vi "FPGA_DMA_Init_5782.vi"(8 "error in (no error)":errorcluster, 11 "FPGA VI Reference":T1) -> (0 "error out":errorcluster, 3 "FPGA VI Out":T1, 5 "Remaining":u32)   [LabVIEW 2013]
uses:
  Config/FPGAref_5782_DMA.ctl
  <vilib>/rvi/interface/common/niFpgaWaitOnOcc.vi
  <vilib>/Utility/error.llb/Error Cluster From Error Code.vi
  <vilib>/rvi/errors/niLvFpgaAdjustHostInterfaceError.vi
  <vilib>/rvi/interface/nirviMethod/nirviMethod.xnode
  <vilib>/rvi/errors/niLvFpgaMergeErrorWithErrorCode.vi
  <vilib>/FPGAPlugInAG/Dynamic/niLvFpga_ReadFifo_Dynamic.vi
  <vilib>/FPGAPlugInAG/Dynamic/niLvFpga_ConfigureFifo_Dynamic.vi
  <vilib>/FPGAPlugInAG/Dynamic/niLvFpga_StartFifo_Dynamic.vi
panel:
  out "Actual Depth":u32
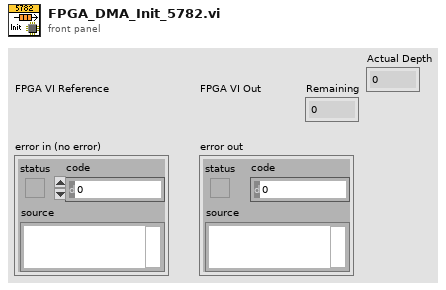
[diagram p1: front panel]
types:
  T1 = typedef "FPGAref_5782_DMA.ctl" = refnum<k20>
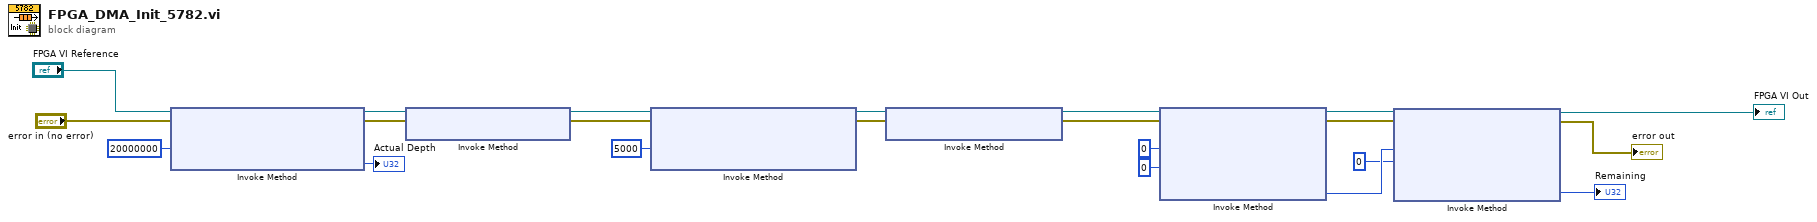
[diagram p0: block diagram]
diagram:
  n1 = xnode "Invoke Method"("FPGA VI Reference In"="FPGA VI Reference", "error in"="error in (no error)", "Requested Depth"=u32 20000000 ("Depth")) -> ("FPGA VI Reference Out"=w18:T1, "error out"=w19:errorcluster, "Actual Depth"=→"Actual Depth":u32)
  n2 = xnode "Invoke Method"("FPGA VI Reference In"=w18, "error in"=w19) -> ("FPGA VI Reference Out"=w7:T1, "error out"=w6:errorcluster)
  n3 = xnode "Invoke Method"("FPGA VI Reference In"=w7, "error in"=w6, "Requested Depth"=u32 5000 ("Depth")) -> ("FPGA VI Reference Out"=w10:T1, "error out"=w9:errorcluster)  [unwired: 1 out]
  n4 = xnode "Invoke Method"("FPGA VI Reference In"=w10, "error in"=w9) -> ("FPGA VI Reference Out"=w4:T1, "error out"=w5:errorcluster)
  n5 = xnode "Invoke Method"("FPGA VI Reference In"=w4, "error in"=w5, "Number of Elements"=u32 0, "Timeout (ms)"=0) -> ("FPGA VI Reference Out"=w13:T1, "error out"=w12:errorcluster, "Elements Remaining"=w15:u32)  [unwired: 1 out]
  n6 = xnode "Invoke Method"("FPGA VI Reference In"=w13, "error in"=w12, "Number of Elements"=w15, "Timeout (ms)"=0) -> ("FPGA VI Reference Out"=→"FPGA VI Out":T1, "error out"=→"error out":errorcluster, "Elements Remaining"=→"Remaining":u32)  [unwired: 1 out]
